vi "Main.vi"() -> ()   [LabVIEW 2019]
doc: "The myRIO Project template acquires acceleration data from the onboard accelerometer and displays the changes of acceleration values in a waveform chart."
uses:
  <vilib>/myRIO/Common/Instrument Driver Framework/myRIO v1.0/UART/vis/myRIO v1.0 Close UART.vi
  <vilib>/myRIO/Common/Instrument Driver Framework/Utilities/vis/FPGA Ref Manager.vi
  <vilib>/myRIO/Common/Instrument Driver Framework/myRIO v1.0/myRIO v1.0 Reset FPGA.vi
  <vilib>/myRIO/Common/Instrument Driver Framework/myRIO v1.0/IRQ/vis/myRIO v1.0 IRQ Info FGV.vi
  <vilib>/myRIO/Common/Instrument Driver Framework/myRIO v1.0/IRQ/vis/myRIO v1.0 Timer IRQ Info FGV.vi
  <vilib>/myRIO/Common/Instrument Driver Framework/myRIO v1.0/IRQ/vis/myRIO v1.0 ISR Agent.vi
  <vilib>/myRIO/Instrument Drivers/Utilities/vis/Reset Index.vi
  <vilib>/myRIO/Common/Instrument Driver Framework/myRIO v1.0/Resource Manager/vis/myRIO v1.0 Block Write Resource Manager.vi
  <vilib>/myRIO/Instrument Drivers/Utilities/Utilities.lvlib
panel:
  in  "Estado_Gripper":bool
  out "Ultrasonido_2":dbl
  out "Ultrasonido_1":dbl
  out "FugaAireDetectada":bool
  in  "U_Velocidad_Angular":dbl min=-3.7 max=3.7 step=0.01
  in  "U_Velocidad_Lineal":dbl min=-0.6 max=0.6 step=0.01
  out "Velocidad_Angular (ENC)":dbl
  out "Velocidad_Lineal (ENC)":dbl
  out "error out":errorcluster
  in  "Stop":bool
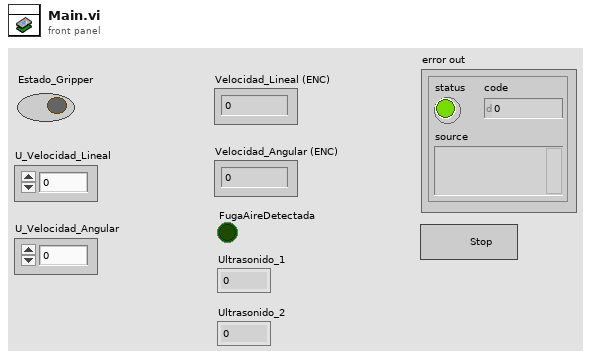
[diagram p1: front panel]
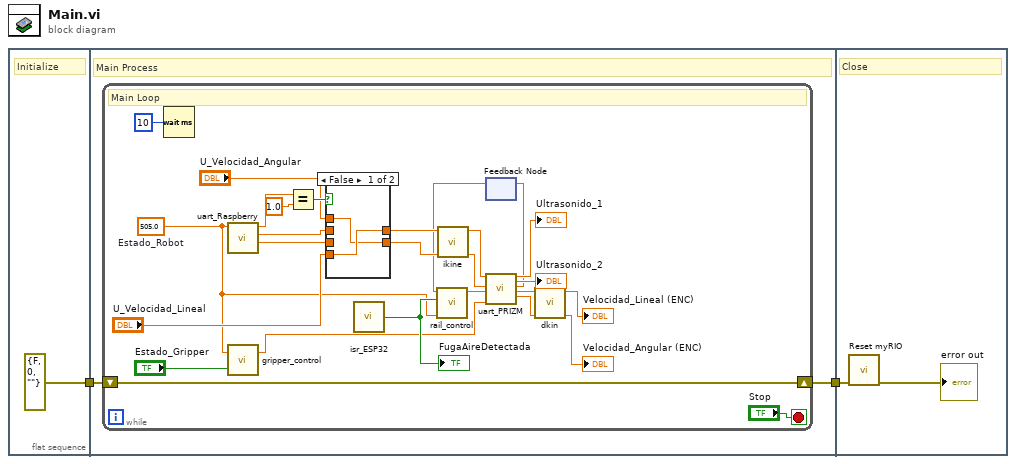
[diagram p0: block diagram]
diagram:
  n1 = flat-sequence {
    tunnel: [errorcluster {"status"=FALSE, "code"=0, "source"=""} ("error in (no error)")] -> w2
    tunnel: w2 -> [w5]
    tunnel: [w4] -> w1
    tunnel: w1 -> [w38]
    frame #0 {
      # "Initialize"
    }
    frame #1 {
      # "Main Process"
      n2 = while {
        shift-right: [w30] -> w4
        shift-left: w5 -> [w30]
        stop <- "Stop" stop-if-true
        w10 = 505.0  # Estado_Robot
        # "Main Loop"
        n3 = Wait (ms)(milliseconds to wait=u32 10) -> ()  [unwired: 1 out]
        n4 = call "uart_Raspberry.vi"("Estado_Robot"=w10) -> ("Velocidad_Angular"=w18:dbl, "Velocidad_Lineal"=w20:dbl, "Peticion_Control"=w22:dbl)  [unwired: 6 in, 2 out]
        n5 = call "gripper_control.vi"("Estado_Gripper"="Estado_Gripper", "Estado_Robot"=w10) -> ("Angulo_Gripper"=w8:dbl)  [unwired: 1 in]
        n6 = Equal?(x=w22, y=1.0) -> (x = y?=w23:bool)
        n7 = case shown="False" w23 {
          tunnel: w20 -> [_ w36]
          tunnel: [w34 w36] -> w19
          tunnel: w18 -> [_ w35]
          tunnel: [w33 w35] -> w17
          tunnel: "U_Velocidad_Lineal" -> [w34 _]
          tunnel: "U_Velocidad_Angular" -> [w33 _]
          frame False {
          }
          frame True {
          }
        }
        n8 = call "isr_ESP32.vi"() -> ("SenalFuga"=w11:bool)  [unwired: 8 in]
        "FugaAireDetectada" <- w11
        n9 = call "ikine.vi"("w"=w17, "v"=w19) -> ("phi_r"=w28:dbl, "phi_d"=w29:dbl)  [unwired: 8 in]
        n10 = feedback #1() -> (w6:dbl)  [unwired: 1 in]
        n11 = call "rail_control.vi"("Medicion_ToF (mm)"=w6, "FugaAire"=w11, "Estado_Robot"=w10) -> ("output (%)"=w14:dbl)  [unwired: 7 in]
        n12 = call "uart_PRIZM.vi"("Motor_Derecho"=w29, "Motor_Izquierdo"=w28, "Motor_Riel"=w14, "Servo_Gripper"=w8) -> ("Ultrasonido_1"=→"Ultrasonido_1":dbl, "Ultrasonido_2"=→"Ultrasonido_2":dbl, "Distancia_ToF"=w7:dbl, "Vel_Derecho"=w27:dbl, "Vel_Izquierdo"=w26:dbl)  [unwired: 9 in, 2 out]
        n13 = feedback-in #1(w7) -> ()
        n14 = call "dkin.vi"("phi_r"=w26, "phi_d"=w27) -> ("w"=→"Velocidad_Angular (ENC)":dbl, "v"=→"Velocidad_Lineal (ENC)":dbl)  [unwired: 8 in]
      }
    }
    frame #2 {
      # "Close"
      n15 = call <vilib>:"Reset myRIO.vi"("error in (no error)"=w38) -> ("error out"=→"error out":errorcluster)  [unwired: 10 in]
    }
  }
